vi "lab3.vi"() -> ()   [LabVIEW 2018]
panel:
  in  "Tab Control":T1(tab)
  in  "E 3":dbl
  in  "Vo":dbl
  in  "R 3":dbl
  in  "c":dbl
  in  "t":dbl
  out "discharge for \ncapacitor":dbl
  in  "Vcc":dbl format="%#_8g"
  in  "Rb1":dbl format="%#_8g"
  in  "Rb2":dbl format="%#_8g"
  in  "RE":dbl format="%#_8g"
  in  "Re":dbl format="%#_8g"
  in  "Rc":dbl format="%#_8g"
  in  "Vin":dbl format="%#_8g"
  in  "RL":dbl format="%#_8g"
  in  "BETA":dbl format="%#_8g"
  out "VB":dbl format="%#_3e"
  out "VE":dbl format="%#_3e"
  out "IE":dbl format="%#_3e"
  out "VC":dbl format="%#_3e"
  out "AV":dbl format="%#_3e"
  out "Vout":dbl format="%#_3e"
  out "Zin":dbl format="%#_3e"
  in  "E":dbl
  in  "R":dbl
  in  "C":dbl
  out "Time Const":dbl
  out "TIME = 0":dbl format="%#_3e"
  out "TIME = 1":dbl format="%#_3e"
  out "TIME = 2":dbl format="%#_3e"
  out "TIME = 3":dbl format="%#_3e"
  out "TIME = 4":dbl format="%#_3e"
  out "TIME = 5":dbl format="%#_3e"
  out "VC T = 0":dbl format="%#_3e"
  out "VC T = 1":dbl format="%#_3e"
  out "VC T = 2":dbl format="%#_3e"
  out "VC T = 3":dbl format="%#_3e"
  out "VC T = 4":dbl format="%#_3e"
  out "VC T = 5":dbl format="%#_3e"
  in  "E 2":dbl
  in  "R 2":dbl
  in  "C 2":dbl
  out "Time Const 2":dbl
  out "TIME = 6":dbl format="%#_3e"
  out "TIME = 7":dbl format="%#_3e"
  out "TIME = 8":dbl format="%#_3e"
  out "TIME = 9":dbl format="%#_3e"
  out "TIME = 10":dbl format="%#_3e"
  out "TIME = 11":dbl format="%#_3e"
  out "VC T = 6":dbl format="%#_3e"
  out "VC T = 7":dbl format="%#_3e"
  out "VC T = 8":dbl format="%#_3e"
  out "VC T = 9":dbl format="%#_3e"
  out "VC T = 10":dbl format="%#_3e"
  out "VC T = 11":dbl format="%#_3e"
  in  "V1":dbl
  in  "V1 angle":dbl
  in  "R1":dbl
  in  "C1":dbl
  in  "L1":dbl
  out "Zt":dbl
  out "Zt angle":dbl
  out "I":dbl
  out "I angle":dbl
  out "Vr":dbl
  out "Vr angle":dbl
  out "Vl":dbl
  out "Vl angle":dbl
  in  "stop":bool
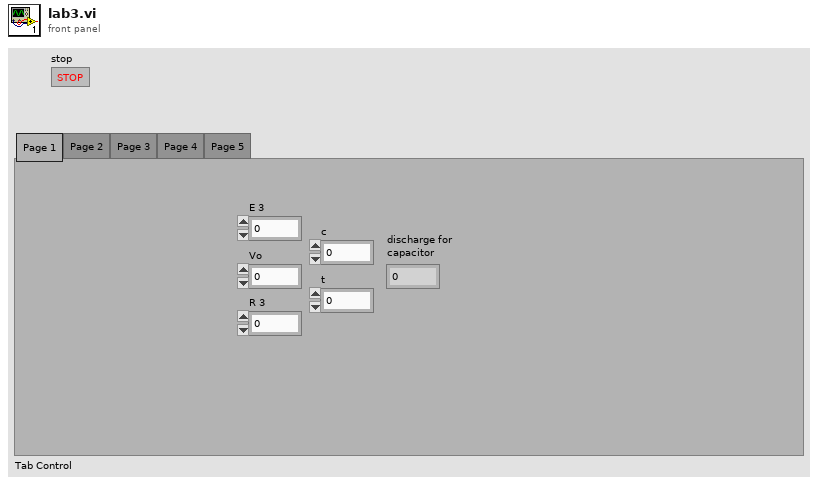
[diagram p1: front panel]
types:
  T1 = enum32{"Page 1", "Page 2", "Page 3", "Page 4", "Page 5"}
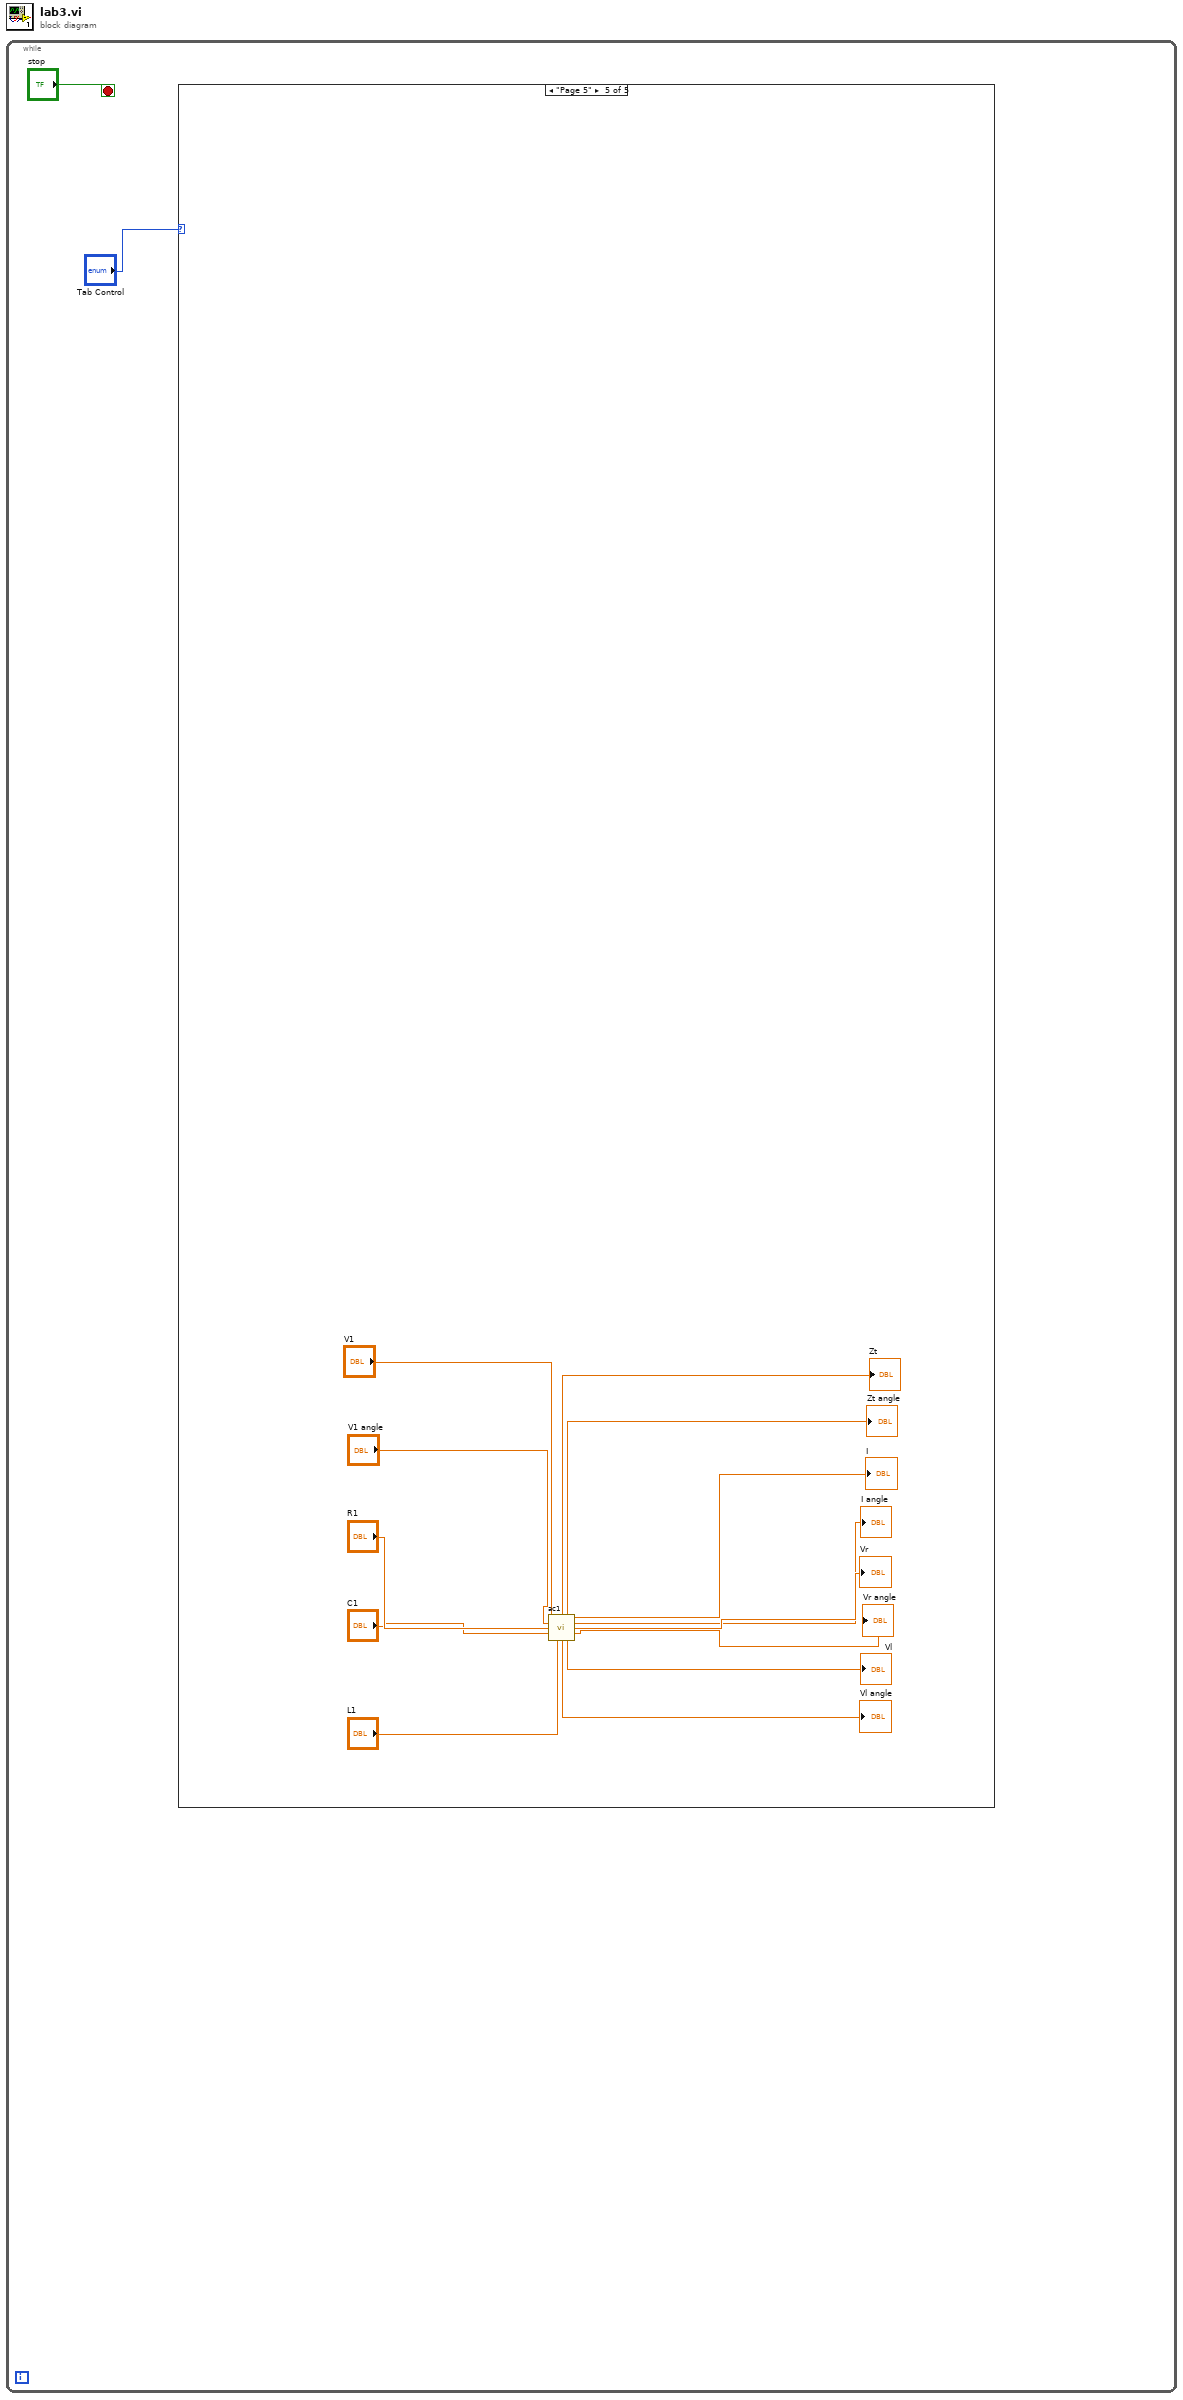
[diagram p0: block diagram]
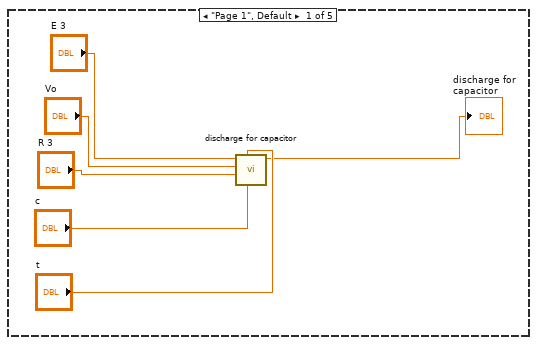
[diagram p2: hidden frame]
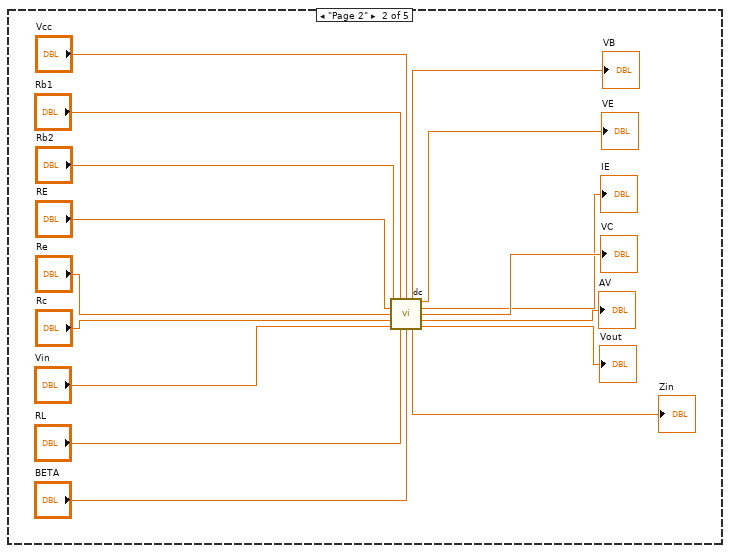
[diagram p3: hidden frame]
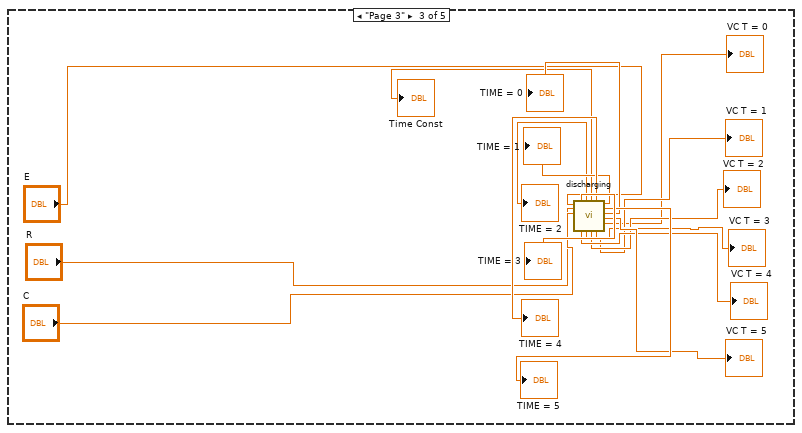
[diagram p4: hidden frame]
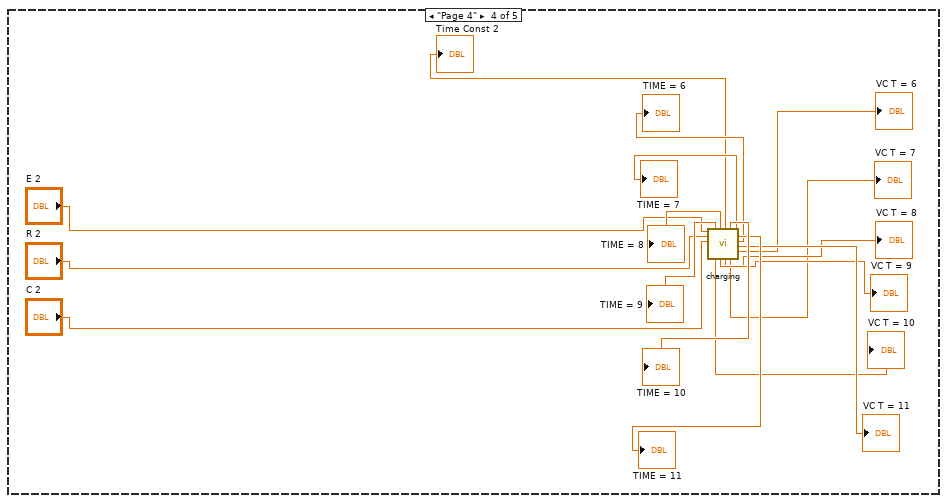
[diagram p5: hidden frame]
diagram:
  n1 = while {
    stop <- "stop" stop-if-true
    n2 = case shown="\"Page 5\"" "Tab Control" {
      frame "Page 1", Default {
        n3 = call "discharge for capacitor.vi"("c"="c", "t"="t", "R"="R 3", "Vo"="Vo", "E"="E 3") -> ("discharge for \ncapacitor"=→"discharge for \ncapacitor":dbl)  [unwired: 6 in]
      }
      frame "Page 2" {
        n4 = call "dc.vi"("Rb2"="Rb2", "Rb1"="Rb1", "Vcc"="Vcc", "RE"="RE", "Re"="Re", "Rc"="Rc", "Vin"="Vin", "RL"="RL", "BETA"="BETA") -> ("VB"=→"VB":dbl, "VE"=→"VE":dbl, "IE"=→"IE":dbl, "VC"=→"VC":dbl, "AV"=→"AV":dbl, "Zin"=→"Zin":dbl, "Vout"=→"Vout":dbl)
      }
      frame "Page 3" {
        n5 = call "discharging.vi"("E"="E", "R"="R", "C"="C") -> ("TIME = 3"=→"TIME = 3":dbl, "VC T = 4"=→"VC T = 4":dbl, "TIME = 2"=→"TIME = 2":dbl, "VC T = 3"=→"VC T = 3":dbl, "Time Const"=→"Time Const":dbl, "VC T = 2"=→"VC T = 2":dbl, "TIME = 4"=→"TIME = 4":dbl, "VC T = 1"=→"VC T = 1":dbl, "TIME = 1"=→"TIME = 1":dbl, "TIME = 5"=→"TIME = 5":dbl, "TIME = 0"=→"TIME = 0":dbl, "VC T = 5"=→"VC T = 5":dbl, "VC T = 0"=→"VC T = 0":dbl)  [unwired: 4 in]
      }
      frame "Page 4" {
        n6 = call "charging.vi"("E in"="E 2", "R in"="R 2", "C in"="C 2") -> ("TIME = 9"=→"TIME = 9":dbl, "VC T = 10"=→"VC T = 10":dbl, "TIME = 8"=→"TIME = 8":dbl, "VC T = 9"=→"VC T = 9":dbl, "Time Const 2"=→"Time Const 2":dbl, "VC T = 8"=→"VC T = 8":dbl, "TIME = 10"=→"TIME = 10":dbl, "VC T = 7"=→"VC T = 7":dbl, "TIME = 7"=→"TIME = 7":dbl, "TIME = 11"=→"TIME = 11":dbl, "TIME = 6"=→"TIME = 6":dbl, "VC T = 11"=→"VC T = 11":dbl, "VC T = 6"=→"VC T = 6":dbl)  [unwired: 4 in]
      }
      frame "Page 5" {
        n7 = call "ac1.vi"("V1"="V1", "V1 angle"="V1 angle", "R1"="R1", "C1"="C1", "L1"="L1") -> ("Zt"=→"Zt":dbl, "Zt angle"=→"Zt angle":dbl, "I"=→"I":dbl, "I angle"=→"I angle":dbl, "Vr"=→"Vr":dbl, "Vr angle"=→"Vr angle":dbl, "Vl angle"=→"Vl angle":dbl, "Vl"=→"Vl":dbl)  [unwired: 3 in]
      }
    }
  }
